vi "P9.vi"() -> ()   [LabVIEW 2018]
uses:
  <vilib>/vision/NI_Vision_Development_Module.lvlib
panel:
  in  "Browser Info":T1={"Browser Size"={"X"=256, "Y"=256}, "Images per Line"=4, "Background Color"=10066329, "Frame Size"=7, "Frame Style"=enum."Step"}
  in  "error in (no error)":errorcluster
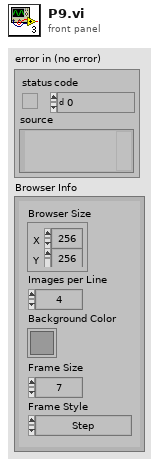
[diagram p1: front panel]
types:
  T1 = cluster{"Browser Size":cluster{"X":i32, "Y":i32}, "Images per Line":i32, "Background Color":u32, "Frame Size":i32, "Frame Style":enum16{"Raised", "Bevelled", "Outline", "Hidden", "Step", "Raised Outline"}}
  T2 = typedef "Image Type" = u32
  T3 = typedef "IMAQ Image.ctl" = refnum<image>
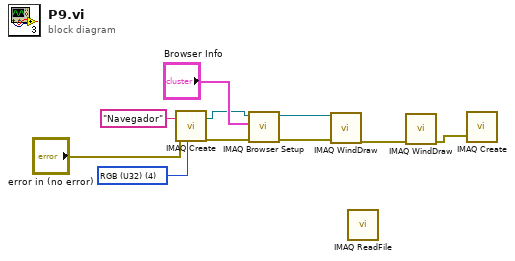
[diagram p0: block diagram]
diagram:
  w10 = T2 4 items=["Grayscale (U8)", "Grayscale (I16)", "Grayscale (SGL)", "Complex (CSG)", "RGB (U32)", "HSL (U32)", "RGB (U64)", "Grayscale (U16)"] ("Image Type")
  n1 = call "IMAQ Create"("Image Name"="Navegador", "Image Type"=w10, "error in (no error)"="error in (no error)") -> ("New Image"=w6:T3, "error out"=w5:errorcluster)  [unwired: 2 in]
  n2 = call "IMAQ Browser Setup"("error in (no error)"=w5, "Browser Info"="Browser Info", "Image In"=w6) -> ("error out"=w4:errorcluster, "Image Browser Out"=w3:T3)  [unwired: 1 in, 2 out]
  n3 = call "IMAQ WindDraw"("error in (no error)"=w4, "Image"=w3) -> ("error out"=w1:errorcluster)  [unwired: 8 in, 1 out]
  n4 = call <userlib>:"IMAQ ReadFile.vi"() -> ()  [unwired: 7 in, 5 out]
  n5 = call "IMAQ WindDraw"("error in (no error)"=w1) -> ("error out"=w2:errorcluster)  [unwired: 9 in, 1 out]
  n6 = call "IMAQ Create"("error in (no error)"=w2) -> ()  [unwired: 4 in, 2 out]
